vi "WriteData.vi"   [LabVIEW 2017, in "NI_ExcelFile.lvlib"]
doc: "Logs data to a temporary location or to the memory. This VI does not write the data to a physical file. If the stream mode of the Create VI is File, the WriteData VI logs the data to the datalog. If the stream mode of the Create VI is Memory, the WriteData VI logs the data to memory. After you log the data, you can use the WriteFile VI to write the data to the actual .xlsx file.\n\n \nExcel refnum: Specifies a reference to the .xlsx file on which to perform the operation. Use the Create VI to create or open the refnum.\n\ndata: Specifies the data you want to write to the .xlsx file.\n\noperation: Specifies the operation you want to perform.\n0 create - Creates a new column in the .xlsx file.\n1 append values - Append input data after a specified channel.\n2 replace all values - Replace all values with input data at a specified channel.\n3 replace value at index - Replace values with input data at a specified channel and index.\n\nchannel index: Specifies the index of the channel you want to configure.\n\nvalue index: Specifies the index of the value you want to append or replace.\n\nerror in: describes error conditions that occur before this node runs. This input provides standard error in functionality.\n\nExcel refnum out: Returns a Microsoft Excel file reference to the .xlsx file on which you performed the operation.\n\nerror out: contains error information. This output provides standard error out functionality."
uses:
  <vilib>/express/express shared/NI_ExcelFile/NI_ExcelFile.lvlib
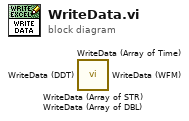
[diagram p0: block diagram]
diagram:
  n1 = call <vilib>:"WriteData (Array of STR).vi"() -> ()  [unwired: 10 in, 2 out]
  n2 = call <vilib>:"WriteData (Array of Time).vi"() -> ()  [unwired: 10 in, 2 out]
  n3 = call <vilib>:"WriteData (DDT).vi"() -> ()  [unwired: 10 in, 2 out]
  n4 = call <vilib>:"WriteData (WFM).vi"() -> ()  [unwired: 10 in, 2 out]
  n5 = call <vilib>:"WriteData (Array of DBL).vi"() -> ()  [unwired: 10 in, 2 out]
